vi "Find.vi"(7 "default":refnum<class "Component Configurations.lvclass">, 8 "error in (no error)":errorcluster, 11 "objects":refnum<class>[](array[class])) -> (0 "error out":errorcluster, 1 "found?":bool, 2 "index":i32, 3 "Component Configurations":refnum<class "Component Configurations.lvclass">)   [LabVIEW 2017, in "DSF Core.lvlib" / "Component Configurations.lvclass"]
uses:
  Component Configurations.lvclass
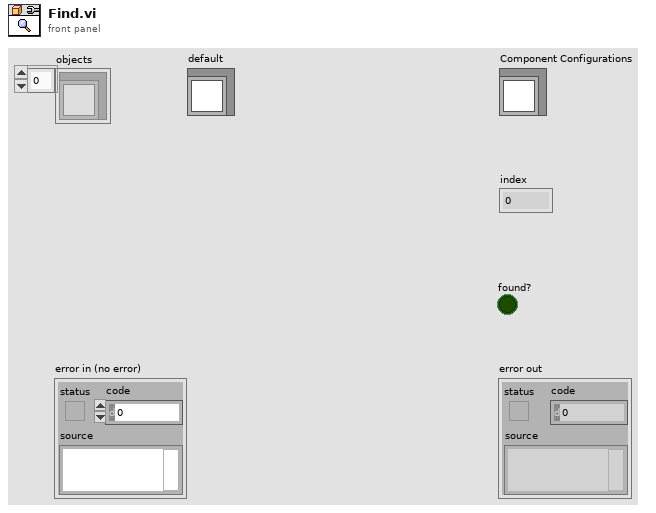
[diagram p1: front panel]
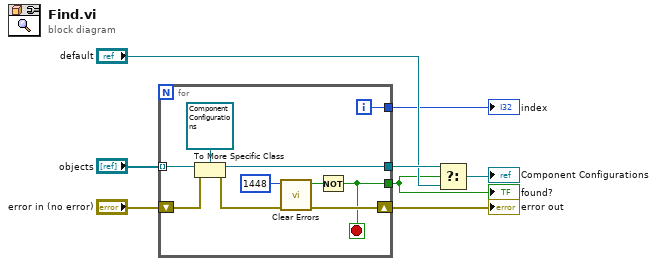
[diagram p0: block diagram]
diagram:
  n1 = for {
    tunnel: "objects" -> [w18] mode=indexing
    shift-right: [w15] -> w7
    shift-left: "error in (no error)" -> [w14]
    tunnel: [w12] -> w2
    tunnel: [w11] -> w5
    tunnel: [w9] -> w1
    i -> [w9]
    stop <- w12 stop-if-true
    n2 = To More Specific Class(target class=refnum<class "Component Configurations.lvclass"> refnum ("Component Configurations out"), reference=w18, error in=w14) -> (specific class reference=w11:refnum<class "Component Configurations.lvclass">, error out=w16:errorcluster)
    n3 = call <vilib>:"Clear Errors.vi"("error in (no error)"=w16, "specific error code to clear (0: all)"=1448) -> ("error out"=w15:errorcluster, "specific error cleared?"=w13:bool)  [unwired: 4 in]
    n4 = Not(x=w13) -> (.not. x?=w12:bool)
  }
  "error out" <- w7
  "found?" <- w2
  "index" <- w1
  n5 = Select(t=w5, s=w2, f="default") -> (s? t:f=→"Component Configurations":refnum<class "Component Configurations.lvclass">)
